vi "calcParity.vi"(1 "Number":u16) -> (0 "Parity":u16)   [LabVIEW 2019]
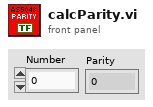
[diagram p1: front panel]
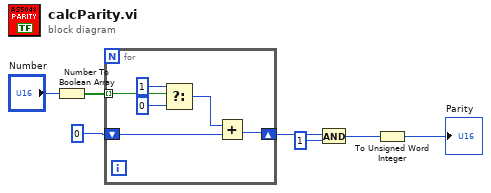
[diagram p0: block diagram]
diagram:
  n1 = Number To Boolean Array(number="Number") -> (Boolean array=w6:bool[])
  n2 = for {
    tunnel: w6 -> [w13] mode=indexing
    shift-right: [w9] -> w4
    shift-left: u8 0 ("f") -> [w8]
    n3 = Select(t=u8 1, s=w13, f=u8 0) -> (s? t:f=w10:u8)
    n4 = Add(x=w10, y=w8) -> (x+y=w9:u8)
  }
  n5 = And(x=w4, y=u8 1) -> (x .and. y?=w2:u8)
  n6 = To Unsigned Word Integer(number=w2) -> (unsigned 16bit integer=→"Parity":u16)
